vi "KG get pump control.vi"(8 "Fehler (Eingang, kein Fehler)":errorcluster, 11 "VISA-Ressourcenname":refnum<visa-resource-name>) -> (0 "Fehler (Ausgang)":errorcluster, 1 "Kommando gesendet":string, 2 "control mode":dbl, 3 "VISA-Ressourcenname (Ausgang)":refnum<visa-resource-name>)   [LabVIEW 2020, in "Linearisierung v2.lvlib" / "Gasteiler.lvlib" / "HovaCAL_Interface.lvlib" / "KGN.lvlib" / "get.lvlib"]
uses:
  get.lvlib
  KGN.lvlib
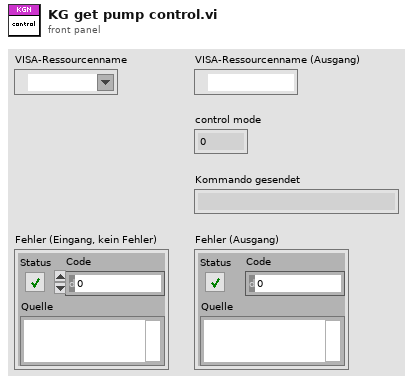
[diagram p1: front panel]
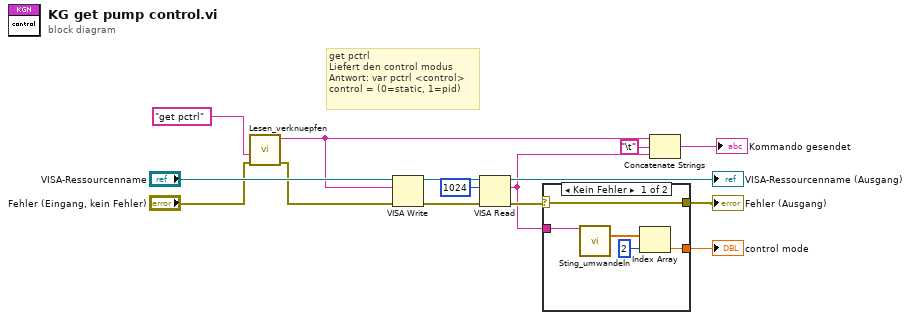
[diagram p0: block diagram]
diagram:
  # "get pctrl\nLiefert den control modus\nAntwort: var pctrl <control>\ncontrol = (0=static, 1=pid)"
  n1 = call "Lesen_verknuepfen.vi"("error in (no error)"="Fehler (Eingang, kein Fehler)", "Order"="get pctrl" ("Schreibpuffer")) -> ("error out"=w9:errorcluster, "Verknüpfter String"=w8:string)  [unwired: 8 in]
  n2 = VISA Write(VISA resource name="VISA-Ressourcenname", write buffer=w8, error in (no error)=w9) -> (VISA resource name out=w15:refnum<visa-resource-name>, error out=w14:errorcluster)  [unwired: 1 out]
  n3 = VISA Read(VISA resource name=w15, byte count=u32 1024 ("Byte-Anzahl"), error in (no error)=w14) -> (VISA resource name out=→"VISA-Ressourcenname (Ausgang)":refnum<visa-resource-name>, read buffer=w2:string, error out=w5:errorcluster)  [unwired: 1 out]
  n4 = case shown="Kein Fehler" w5 {
    selector: w5 -> [w16 _]
    tunnel: w2 -> [w20 _]
    tunnel: [w17 _] -> w6
    tunnel: [w16 _] -> w4
    frame No Error {
      n5 = call "Sting_umwandeln.vi"("Lesepuffer"=w20) -> ("Zahl array"=w18:dbl[])  [unwired: 8 in, 6 out]
      n6 = Index Array(array=w18, index=2 ("Index")) -> (element=w17:dbl)
    }
    frame Error {
    }
  }
  "Fehler (Ausgang)" <- w4
  "control mode" <- w6
  n7 = Concatenate Strings(w8, "\t", w2) -> (→"Kommando gesendet":string)
